vi "test-cubic-spline-01.vi"() -> (3 "Test Passed":bool)   [LabVIEW 2019]
uses:
  <vilib>/Rock Robotics/WPI/ThirdParty/JAS_Junk/TrajLib/POSEwCURVATURE.ctl
  <vilib>/Rock Robotics/WPI/ThirdParty/JAS_Junk/TrajLib/POSE2D.ctl
  <vilib>/Rock Robotics/WPI/ThirdParty/JAS_Junk/TrajLib/TRANSLATION2D.ctl
  <vilib>/Rock Robotics/WPI/ThirdParty/JAS_Junk/TrajLib/ROTATION2D.ctl
  <vilib>/Rock Robotics/WPI/ThirdParty/JAS_Junk/TrajLib/Rotation_CreateAngle.vi
  <vilib>/Rock Robotics/WPI/ThirdParty/JAS_Junk/TrajLib/Util_CalcDist.vi
  <vilib>/Rock Robotics/WPI/ThirdParty/JAS_Junk/TrajLib/Trajectory_Library.lvlib
panel:
  out "XY Graph":cluster{dbl[], dbl[]}(graph)
  out "All Interior \nwayPoints\nFound (True)":bool
  out "end rot = 0":dbl
  out "end y = 0":dbl
  out "end x = 0":dbl
  out "start rot = 0":dbl
  out "start y = 0":dbl
  out "start x = 0":dbl
  out "max dtheta < 0.0872":dbl
  out "max dy < 0.00127":dbl
  out "max dx  < 0.127":dbl
  out "Overall Error":errorcluster
  out "Elements":i32
  out "Create Spline Error":errorcluster
  out "SplinePoses\nWCurve":T1[](array[typedef]) {"POSE"."ROTATION"."SIN" format="%13.4f"; "POSE"."ROTATION"."COS" format="%13.4f"; "POSE"."ROTATION"."VALUE" format="%13.4f"; "POSE"."TRANSLATION"."Y" format="%14.3f"; "POSE"."TRANSLATION"."X" format="%14.3f"}
  out "Elapsed Time":dbl
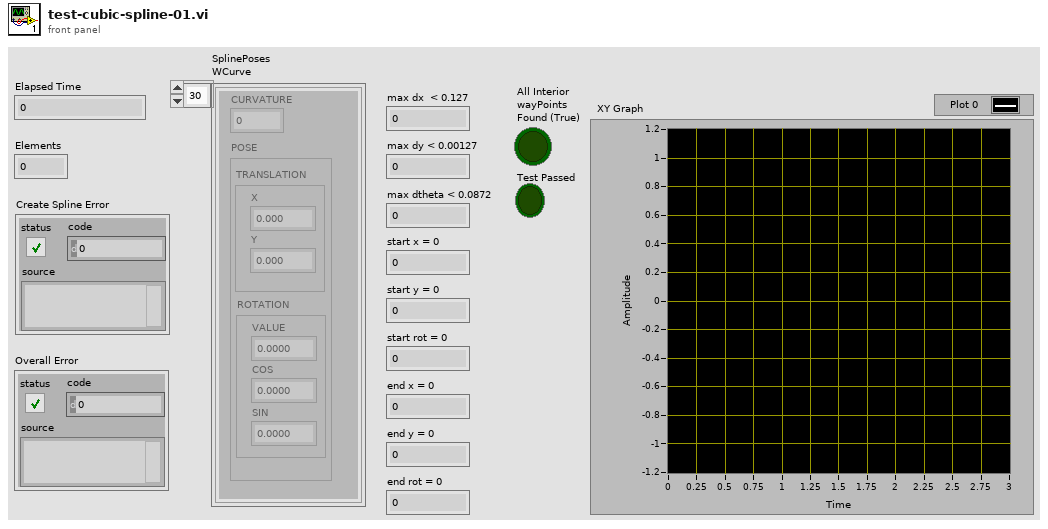
[diagram p1: front panel]
types:
  T1 = typedef "Trajectory_Library.lvlib/POSEwCURVATURE.ctl" = cluster{"CURVATURE":dbl, "POSE":T2}
  T2 = typedef "Trajectory_Library.lvlib/POSE2D.ctl" = cluster{"TRANSLATION":T3, "ROTATION":T4}
  T3 = typedef "Trajectory_Library.lvlib/TRANSLATION2D.ctl" = cluster{"X":dbl, "Y":dbl}
  T4 = typedef "Trajectory_Library.lvlib/ROTATION2D.ctl" = cluster{"VALUE":dbl, "COS":dbl, "SIN":dbl}
  T5 = typedef "Trajectory_Library.lvlib/SPLINE_CTRL_VECTOR.ctl" = cluster{"Xs":dbl[], "Ys":dbl[]}
  T6 = typedef "Trajectory_Library.lvlib/SPLINE.ctl" = cluster{"Degree":i32, "Coefficients":T7}
  T7 = typedef "NI_Matrix.lvlib/RealMatrix.ctl" = dbl[][]
  T8 = typedef "Trajectory_Library.lvlib/TWIST2D.ctl" = cluster{"dX":dbl, "dY":dbl, "dTHETA":dbl}
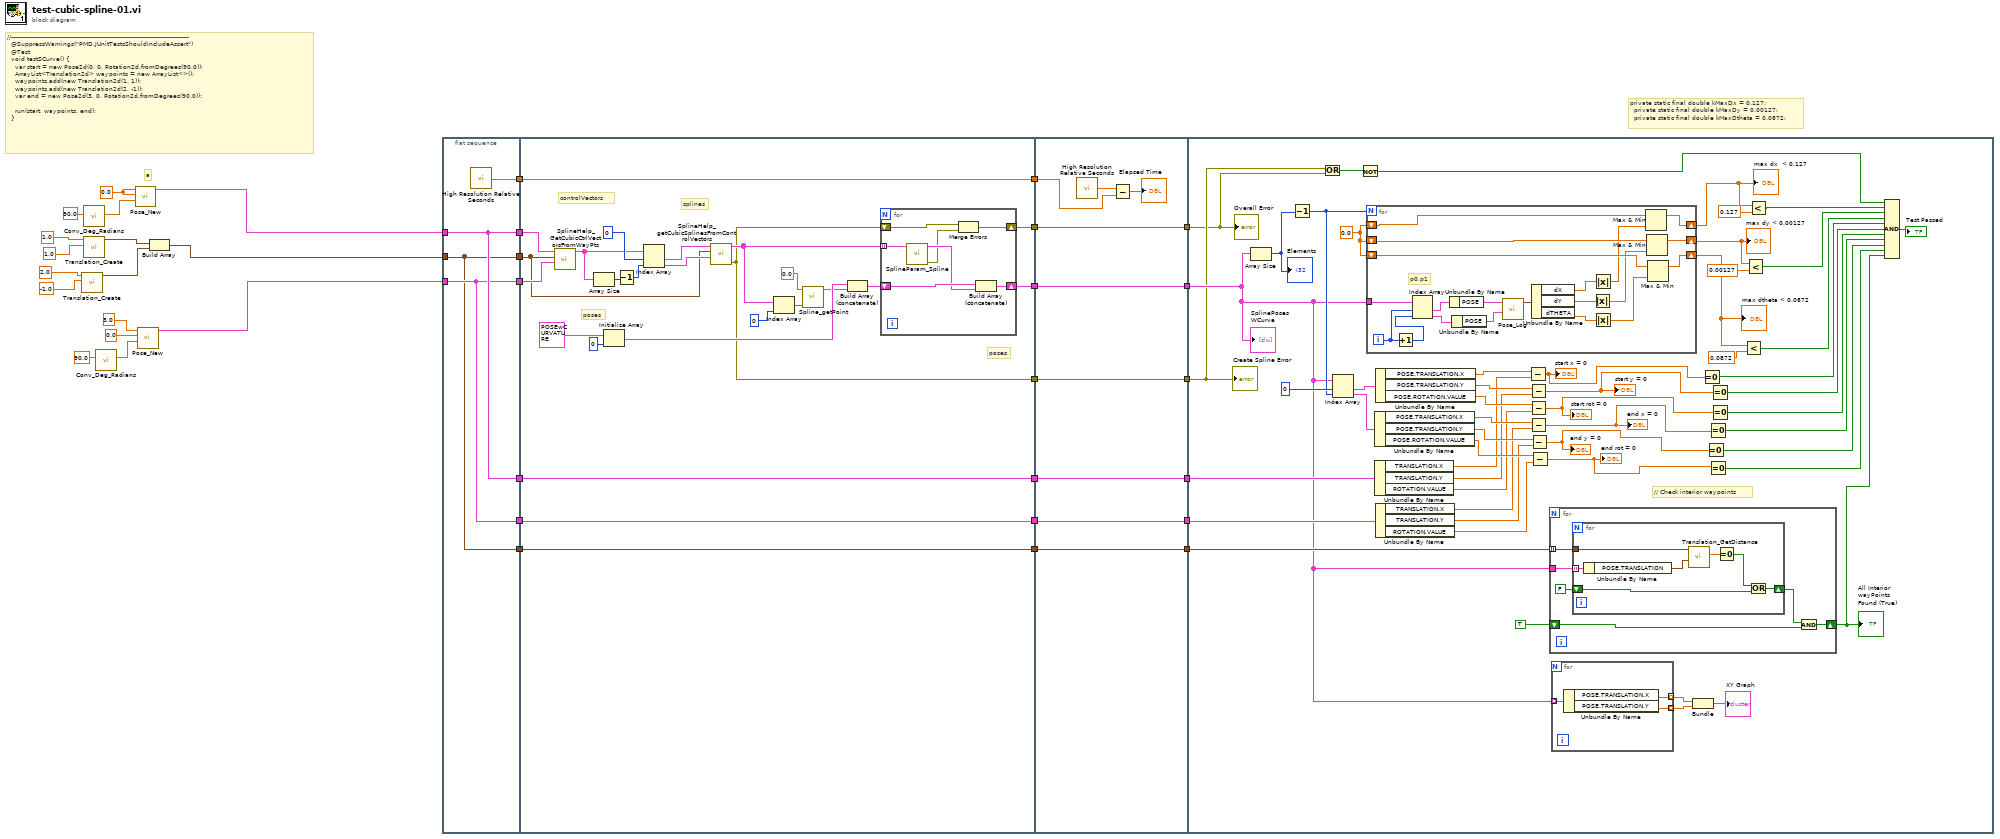
[diagram p0: block diagram]
diagram:
  w14 = 0.0 ("X")
  # "a"
  # "//-----------------------------------------------------------------------------------------\n  @SuppressWarnings(\"PMD.JUnitTestsShouldIncludeAssert\")\n  @Test\n  void testSCurve() {\n    var start = new Pose2d(0, 0, Rotation2d.fromDegrees(90.0));\n    ArrayList<Translation2d> waypoints = new ArrayList<>();\n    waypoints.add(new Translation2d(1, 1));\n    waypoints.add(new Translation2d(2, -1));\n    var end = new Pose2d(3, 0, Rotation2d.fromDegrees(90.0));\n\n    run(start, waypoints, end);\n  }"
  # "private static final double kMaxDx = 0.127;\n  private static final double kMaxDy = 0.00127;\n  private static final double kMaxDtheta = 0.0872;"
  n1 = call <vilib>:"Translation_Create.vi"("Y"=-1.0, "X"=2.0) -> ("TRANSLATION"=w10:T3)  [unwired: 9 in]
  n2 = call <vilib>:"Conv_Deg_Radians.vi"("Degress"=90.0) -> ("Radians"=w13:dbl)  [unwired: 10 in]
  n3 = call <vilib>:"Translation_Create.vi"("Y"=1.0, "X"=1.0) -> ("TRANSLATION"=w11:T3)  [unwired: 9 in]
  n4 = call <vilib>:"Conv_Deg_Radians.vi"("Degress"=90.0) -> ("Radians"=w4:dbl)  [unwired: 10 in]
  n5 = call <vilib>:"Pose_New.vi"("Heading"=w13, "Y"=w14, "X"=w14) -> ("out POSe"=w3:T2)  [unwired: 8 in]
  n6 = call <vilib>:"Pose_New.vi"("Heading"=w4, "Y"=0.0, "X"=3.0) -> ("out POSe"=w1:T2)  [unwired: 8 in]
  n7 = Build Array(w11, w10) -> (w2:T3[])
  n8 = flat-sequence {
    tunnel: w3 -> [w39]
    tunnel: [w39] -> w36
    tunnel: w2 -> [w37]
    tunnel: [w37] -> w35
    tunnel: w1 -> [w38]
    tunnel: [w38] -> w34
    tunnel: [w40] -> w33
    tunnel: [w39] -> w25
    tunnel: [w38] -> w22
    tunnel: [w37] -> w17
    tunnel: w36 -> [w65]
    tunnel: w35 -> [w57]
    tunnel: w34 -> [w64]
    tunnel: [w56] -> w32
    tunnel: w33 -> [w56]
    tunnel: [w46] -> w31
    tunnel: [w45] -> w29
    tunnel: [w44] -> w27
    tunnel: w25 -> [w43]
    tunnel: [w43] -> w24
    tunnel: w22 -> [w42]
    tunnel: [w42] -> w21
    tunnel: [w41] -> w18
    tunnel: w17 -> [w41]
    tunnel: w32 -> [w81]
    tunnel: w31 -> [w80]
    tunnel: [w80] -> w30
    tunnel: w29 -> [w79]
    tunnel: [w79] -> w28
    tunnel: w27 -> [w78]
    tunnel: [w78] -> w26
    tunnel: w24 -> [w75]
    tunnel: [w75] -> w23
    tunnel: w21 -> [w74]
    tunnel: [w74] -> w20
    tunnel: [w73] -> w19
    tunnel: w18 -> [w73]
    tunnel: w30 -> [w109]
    tunnel: w28 -> [w84]
    tunnel: w26 -> [w83]
    tunnel: w23 -> [w132]
    tunnel: w20 -> [w131]
    tunnel: w19 -> [w114]
    frame #0 {
      n9 = call <vilib>:"High Resolution Relative Seconds.vi"() -> ("relative seconds"=w40:dbl)
    }
    frame #1 {
      # "poses"
      # "poses"
      # "splines"
      # "controlVectors"
      n10 = call <vilib>:"SplineHelp_GetCubicCtrlVectorsFromWayPts.vi"("Enging POSE"=w64, "Interior WAYPOINTS"=w57, "Starting POSE"=w65) -> ("SplineControlVectors"=w61:T5[])  [unwired: 8 in]
      n11 = Array Size(array=w61) -> (size(s)=w62:i32)
      n12 = Initialize Array(T1 {"CURVATURE"=0.0, "POSE"={"TRANSLATION"={"X"=0.0, "Y"=0.0}, "ROTATION"={"VALUE"=0.0, "COS"=1.0, "SIN"=0.0}}} ("POSEwCURVATURE"), 0 ("dimension size")) -> (w50:T1[])
      n13 = Decrement(x=w62) -> (x-1=w60:i32)
      n14 = Index Array(array=w61, index #1=0 ("index"), index #2=w60) -> (element #1=w59:T5, element #2=w58:T5)
      n15 = call <vilib>:"SplineHelp_getCubicSplinesFromControlVectors.vi"("endCtrlVector"=w58, "InternalWaypoints"=w57, "startCtrlVector"=w59) -> ("error out"=w45:errorcluster, "splines"=w47:T6[])  [unwired: 3 in, 4 out]
      n16 = Index Array(array=w47, index=0) -> (element=w52:T6)
      n17 = call <vilib>:"Spline_getPoint.vi"("inputSPLINE"=w52, "Time"=0.0) -> ("POSEwCURVATURE"=w49:T1)  [unwired: 9 in]
      n18 = Build Array (concatenate)(w50, w49) -> (w48:T1[])
      n19 = for {
        shift-right: [w69] -> w46
        shift-left: w48 -> [w71]
        tunnel: w47 -> [w72] mode=indexing
        shift-right: [w67] -> w44
        shift-left: w45 -> [w68]
        n20 = call <vilib>:"SplineParam_Spline.vi"("inputSPLINE"=w72) -> ("error out"=w66:errorcluster, "outputPOSEwCURVATURE"=w70:T1[])  [unwired: 9 in]
        n21 = Merge Errors(w68, w66) -> (w67:errorcluster)
        n22 = Build Array (concatenate)(w71, w70) -> (w69:T1[])
      }
    }
    frame #2 {
      n23 = call <vilib>:"High Resolution Relative Seconds.vi"() -> ("relative seconds"=w76:dbl)
      n24 = Subtract(x=w76, y=w81) -> (x-y=→"Elapsed Time":dbl)
    }
    frame #3 {
      w133 = 0.0
      # "// Check interior waypoints"
      n25 = Array Size(array=w109) -> (size(s)=w134:i32)
      "Elements" <- w134
      n26 = Decrement(x=w134) -> (x-1=w129:i32)
      n27 = Or(x=w84, y=w83) -> (x .or. y?=w85:bool)
      n28 = Index Array(array=w109, index #1=0 ("index"), index #2=w129) -> (element #1=w128:T1, element #2=w127:T1)
      n29 = Not(x=w85) -> (.not. x?=w82:bool)
      n30 = for {
        N: w129 -> [_]
        tunnel: w109 -> [w168]
        shift-right: [w159] -> w106
        shift-left: w133 -> [w156]
        shift-right: [w157] -> w108
        shift-left: w133 -> [w154]
        shift-right: [w158] -> w107
        shift-left: w133 -> [w155]
        i -> [w170]
        # "p0,p1"
        n31 = Increment(x=w170) -> (x+1=w169:i32)
        n32 = Index Array(array=w168, index #1=w170, index #2=w169) -> (element #1=w167:T1, element #2=w166:T1)
        n33 = Unbundle By Name(w167) -> ("POSE"=w165:T2)
        n34 = Unbundle By Name(w166) -> ("POSE"=w164:T2)
        n35 = call <vilib>:"Pose_Log.vi"("end POSE"=w164, "in POSE"=w165) -> ("out TWIST"=w163:T8)  [unwired: 9 in]
        n36 = Unbundle By Name(w163) -> ("dX"=w160:dbl, "dY"=w161:dbl, "dTHETA"=w162:dbl)
        n37 = Absolute Value(x=w161) -> (abs(x)=w152:dbl)
        n38 = Absolute Value(x=w160) -> (abs(x)=w153:dbl)
        n39 = Absolute Value(x=w162) -> (abs(x)=w151:dbl)
        n40 = Max & Min(x=w156, y=w153) -> (max(x,y)=w159:dbl)  [unwired: 1 out]
        n41 = Max & Min(x=w155, y=w152) -> (max(x,y)=w158:dbl)  [unwired: 1 out]
        n42 = Max & Min(x=w154, y=w151) -> (max(x,y)=w157:dbl)  [unwired: 1 out]
      }
      "max dx  < 0.127" <- w106
      "max dy < 0.00127" <- w107
      "max dtheta < 0.0872" <- w108
      n43 = Unbundle By Name(w127) -> ("POSE.TRANSLATION.X"=w123:dbl, "POSE.TRANSLATION.Y"=w122:dbl, "POSE.ROTATION.VALUE"=w121:dbl)
      n44 = Unbundle By Name(w132) -> ("TRANSLATION.X"=w120:dbl, "TRANSLATION.Y"=w119:dbl, "ROTATION.VALUE"=w118:dbl)
      n45 = Unbundle By Name(w128) -> ("POSE.TRANSLATION.X"=w126:dbl, "POSE.TRANSLATION.Y"=w125:dbl, "POSE.ROTATION.VALUE"=w124:dbl)
      n46 = Unbundle By Name(w131) -> ("TRANSLATION.X"=w117:dbl, "TRANSLATION.Y"=w116:dbl, "ROTATION.VALUE"=w115:dbl)
      n47 = Subtract(x=w126, y=w120) -> (x-y=w99:dbl)
      "start x = 0" <- w99
      n48 = Subtract(x=w125, y=w119) -> (x-y=w98:dbl)
      "start y = 0" <- w98
      n49 = Subtract(x=w124, y=w118) -> (x-y=w97:dbl)
      "start rot = 0" <- w97
      n50 = Subtract(x=w123, y=w117) -> (x-y=w96:dbl)
      "end x = 0" <- w96
      n51 = Subtract(x=w122, y=w116) -> (x-y=w95:dbl)
      "end y = 0" <- w95
      n52 = Subtract(x=w121, y=w115) -> (x-y=w94:dbl)
      "end rot = 0" <- w94
      n53 = for {
        tunnel: w114 -> [w138] mode=indexing
        tunnel: w109 -> [w143]
        shift-right: [w142] -> w87
        shift-left: TRUE -> [w141]
        n54 = for {
          tunnel: w143 -> [w147] mode=indexing
          shift-right: [w150] -> w139
          shift-left: FALSE -> [w149]
          tunnel: w138 -> [w148]
          n55 = Unbundle By Name(w147) -> ("POSE.TRANSLATION"=w146:T3)
          n56 = call <vilib>:"Translation_GetDistance.vi"("other Translation"=w146, "In Translation"=w148) -> ("Distance"=w145:dbl)  [unwired: 9 in]
          n57 = Equal To 0?(x=w145) -> (x = 0?=w144:bool)
          n58 = Or(x=w144, y=w149) -> (x .or. y?=w150:bool)
        }
        n59 = And(x=w139, y=w141) -> (x .and. y?=w142:bool)
      }
      "All Interior \nwayPoints\nFound (True)" <- w87
      n60 = for {
        tunnel: [w137] -> w112 mode=indexing
        tunnel: [w136] -> w111 mode=indexing
        tunnel: w109 -> [w135] mode=indexing
        n61 = Unbundle By Name(w135) -> ("POSE.TRANSLATION.X"=w137:dbl, "POSE.TRANSLATION.Y"=w136:dbl)
      }
      n62 = Bundle(w112, w111) -> (→"XY Graph":cluster{dbl[], dbl[]})  [unwired: 1 in]
      n63 = Equal To 0?(x=w99) -> (x = 0?=w93:bool)
      n64 = Equal To 0?(x=w95) -> (x = 0?=w89:bool)
      n65 = Equal To 0?(x=w96) -> (x = 0?=w90:bool)
      n66 = Equal To 0?(x=w94) -> (x = 0?=w88:bool)
      n67 = Equal To 0?(x=w98) -> (x = 0?=w92:bool)
      n68 = Equal To 0?(x=w97) -> (x = 0?=w91:bool)
      n69 = Less?(x=w108, y=0.0872) -> (x < y?=w100:bool)
      n70 = Less?(x=w107, y=0.00127) -> (x < y?=w101:bool)
      n71 = Less?(x=w106, y=0.127) -> (x < y?=w102:bool)
      n72 = Compound Arithmetic op=AND(w82, w102, w101, w100, w93, w92, w91, w90, w89, w88, w87) -> (→"Test Passed":bool)
      "SplinePoses\nWCurve" <- w109
      "Create Spline Error" <- w84
      "Overall Error" <- w83
    }
  }
